vi "OpenTempEXCEL.vi"(8 "错误输入（无错误）":errorcluster, 11 "路径":path=path "C:/Users/Administrator/Desktop/GRR模板/Test.xlsx") -> (2 "Worksheets":refnum<k7>, 3 "引用输出":refnum<k7>)   [LabVIEW 2017]
panel:
  in  "Excel._Application":refnum<k7>
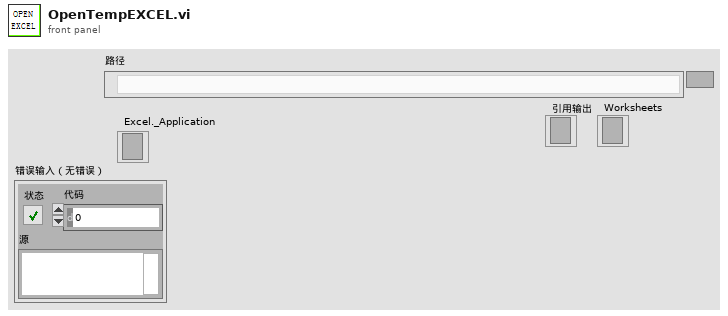
[diagram p1: front panel]
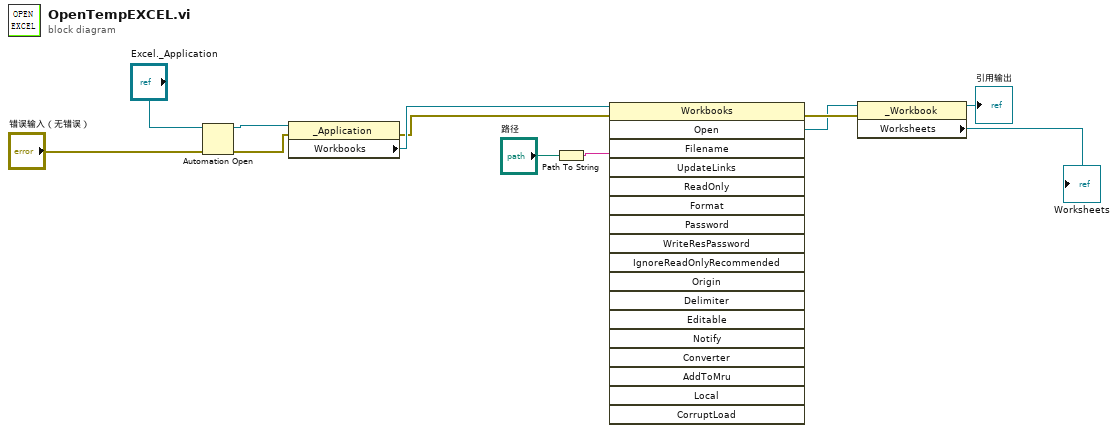
[diagram p0: block diagram]
diagram:
  n1 = Automation Open(error in (no error)="错误输入（无错误）", Automation Refnum="Excel._Application") -> (Automation Refnum=w11:refnum<k7>, error out=w4:errorcluster)  [unwired: 2 in]
  n2 = property on="属性节点" class="_Application"(reference=w11, error in=w4) -> (error out=w7:errorcluster, "Workbooks"=w10:refnum<k7>)  [unwired: 1 out]
  n3 = Path To String(path="路径") -> (string=w8:string)
  n4 = invoke on="调用节点" class="Workbooks" method="Open"(reference=w10, error in=w7, "Filename"=w8) -> (error out=w6:errorcluster, "Open"=w5:refnum<k7>)  [unwired: 15 in, 16 out]
  n5 = property on="属性节点" class="_Workbook"(reference=w5, error in=w6) -> (reference out=→"引用输出":refnum<k7>, "Worksheets"=→"Worksheets":refnum<k7>)  [unwired: 1 out]
